vi "cDLTS progress.vi"(9 "Current sample temperature":dbl[unit], 10 "Tstop":dbl[unit], 11 "Tstart":dbl[unit]) -> (2 "Progress":dbl, 3 "Still not finished":bool)   [LabVIEW 2019]
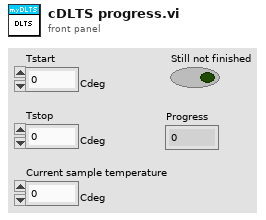
[diagram p1: front panel]
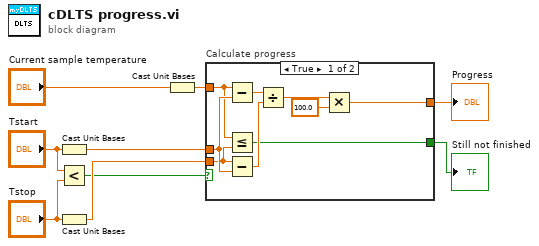
[diagram p0: block diagram]
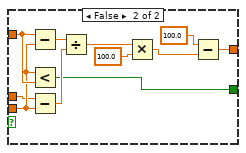
[diagram p2: hidden frame]
diagram:
  n1 = Cast Unit Bases(0:"Tstart") -> (2:w3:dbl)  [unwired: 1 in]
  n2 = Less?(x="Tstart", y="Tstop") -> (x < y?=w1:bool)
  n3 = Cast Unit Bases(0:"Tstop") -> (2:w5:dbl)  [unwired: 1 in]
  n4 = Cast Unit Bases(0:"Current sample temperature") -> (2:w8:dbl)  [unwired: 1 in]
  n5 = case "Calculate progress" shown="True" w1 {
    tunnel: w5 -> [w11 w23]
    tunnel: w8 -> [w12 w25]
    tunnel: w3 -> [w18 w22]
    tunnel: [w13 w19] -> w6
    tunnel: [w10 w24] -> w7
    frame True {
      n6 = Subtract(x=w12, y=w18) -> (x-y=w16:dbl)
      n7 = Less Or Equal?(x=w12, y=w11) -> (x <= y?=w10:bool)
      n8 = Subtract(x=w11, y=w18) -> (x-y=w17:dbl)
      n9 = Divide(x=w16, y=w17) -> (x/y=w15:dbl)
      n10 = Multiply(x=w15, y=100.0) -> (x*y=w13:dbl)
    }
    frame False {
      n11 = Subtract(x=w25, y=w23) -> (x-y=w28:dbl)
      n12 = Less?(x=w23, y=w25) -> (x < y?=w24:bool)
      n13 = Subtract(x=w22, y=w23) -> (x-y=w29:dbl)
      n14 = Divide(x=w28, y=w29) -> (x/y=w27:dbl)
      n15 = Multiply(x=w27, y=100.0) -> (x*y=w21:dbl)
      n16 = Subtract(x=100.0, y=w21) -> (x-y=w19:dbl)
    }
  }
  "Still not finished" <- w7
  "Progress" <- w6
